vi "RetroParse.vi"(11 "Choose Directory":path) -> ()   [LabVIEW 2022 SP3]
panel:
  out "Raw data":i16[][](graph)
  out "Root Name":string
  out "File num":i32
  in  "Use Selected Files":bool
  in  "Listbox":i32[](listbox)
  in  "file ext":string="000"
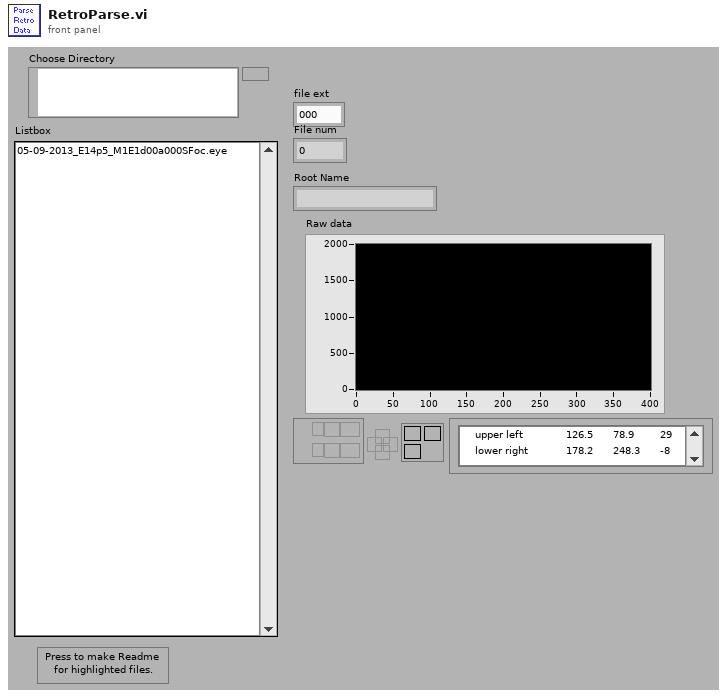
[diagram p1: front panel]
types:
  T1 = enum16{"open", "replace", "create", "open or create", "replace or create", "replace or create with confirmation"}
  T2 = enum16{"big-endian, network order", "native, host order", "little-endian"}
  T3 = typedef "Header.ctl" = cluster{"header info":cluster{"Header":string, "Head length":i16}, "A/D info":cluster{"# rf points per line":u16, "# lines per scan":u16, "sample rate MHz":u16, "# A/D bits":i16, "# bytes per A/D":u16, "TGC Flag":u16, "A/D Type":string}, "Tranducer Info":cluster{"bandwidth":sgl, "center freq":sgl, "start freq":sgl, "ID":i32}, "Scan Info":cluster{"delay":sgl, "pivot distance":sgl, "sector scan angle":sgl, "operator":string, "Scan Mode":string, "location":string}, "Time/Date Info":cluster{"date":string, "time":string}, "RF Info":cluster{"RF file name":string, "RF file att":string, "RF cal file name":string, "RF cal file att":string}, "Patient Info":cluster{"ID":string, "extended ID":string, "age":u16, "sex":string, "previously\nscanned":string, "PSA":sgl, "LOS":u8, "Ethnicty 2":u8, "Race":u8}, "Tissue Type":cluster{"organ":i16, "disease type":i16, "disease location":i16, "IQ_pts":u16, "RcvBuffer":u8, "RcvFrame":u16, "IQBuff":u8, "IQFrame":u16, "IQPage":u8}, "Votage scaling":cluster{"Digitizer (dB)":sgl, "Gain (dB)":sgl, "Atten (dB)":sgl}, "Comment":string, "Misc Info":cluster{"avg num":u16, "c speed":i16, "Div By or SF zones":i16, "XMIT CHS":u8, "RCV CHS":u8, "Xmit angle":sgl}, "Therapy Parameters":cluster{"Theraputic Freq (MHz)":sgl, "Time on (s)":sgl, "Therapy amplitude (mV)":sgl, "Lines Before":u16, "Lines After":u16}, "Scan Settings":cluster{"Energy (uJ or V)":u8, "Damp (Ohm) or Fc":u8, "HP Filt (KHz)":u8, "LP Filt (MHz)":u8, "Gain (db)":u8, "prf (kHz)":sgl, "Distance between\nscan lines (um)":u16, "Distance between\nscan planes (um)":u16, "Scan line gap (um)":sgl, "Scan plane gap (um)":sgl}, "Compression Parameters":cluster{"F1 (MHz)":sgl, "F2 (MHz)":sgl, "% taper":sgl, "duration":sgl}, "Patient Info Xtra":cluster{"First Name":string, "Last Name":string, "Notes":string}, "ROI Box":u16[]}
  T4 = cluster{"Energy (uJ) or V":u8, "Damp (Ohm) or Fc":u8, "HP Filt(KHz) ":u8, "LP Filt (MHz)":u8, "Gain (db)":u8, "prf (kHz)":sgl, "Distance between\nscan lines (mm)":u16, "Distance between\nscan planes (mm)":u16, "Scan line gap (um)":sgl, "Scan plane gap (um)":sgl}
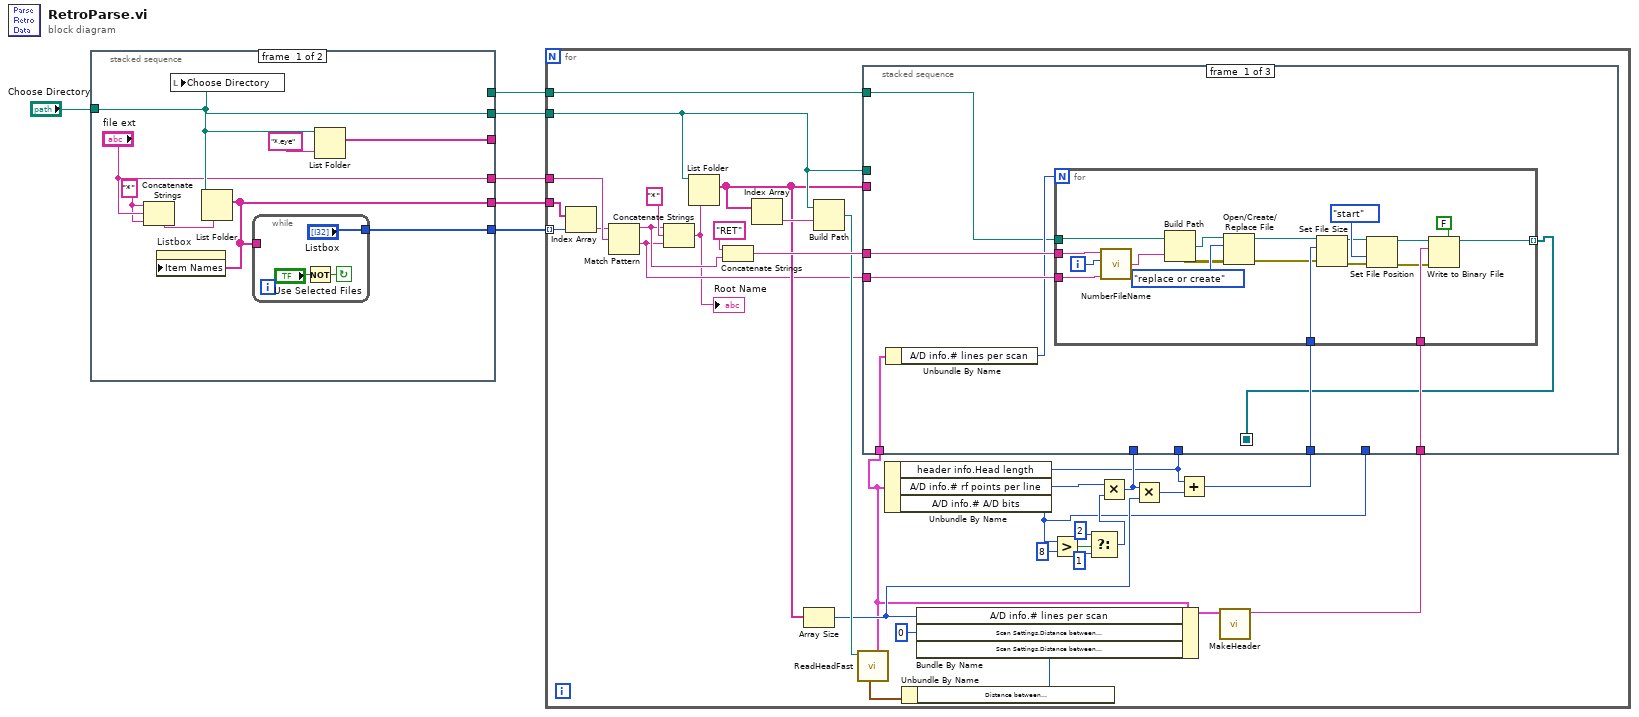
[diagram p0: block diagram]
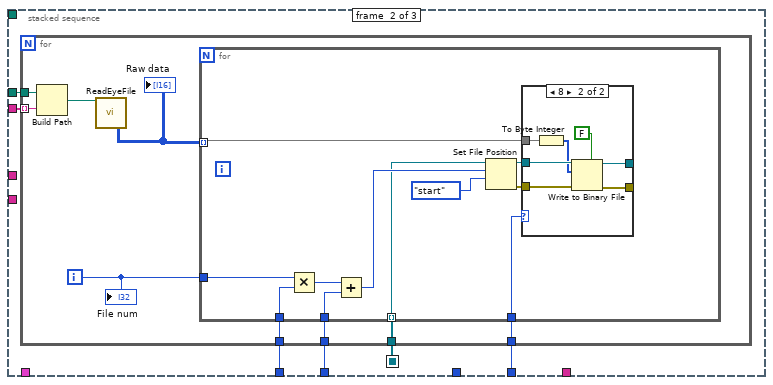
[diagram p2: hidden frame]
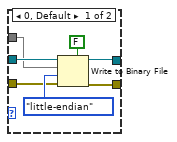
[diagram p3: hidden frame]
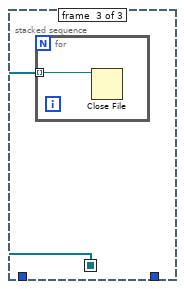
[diagram p4: hidden frame]
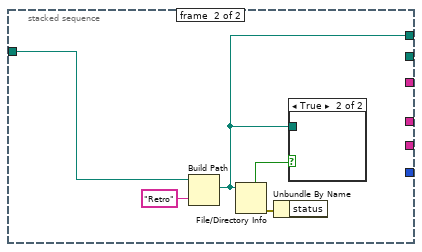
[diagram p5: hidden frame]
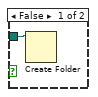
[diagram p6: hidden frame]
diagram:
  n1 = stacked-sequence {
    tunnel: "Choose Directory" -> [w10 w22]
    tunnel: [w13 _] -> _
    tunnel: [w12 _] -> w5
    tunnel: [w11 _] -> w4
    tunnel: ["file ext" _] -> w3
    tunnel: [w10 _] -> w2
    tunnel: [_ w18] -> w1
    frame #0 {
      w7 = "*" ("prompt")
      n2 = Concatenate Strings(w7, "file ext", w7) -> (w8:string)
      n3 = local write "Choose Directory"(w10) -> ()
      n4 = List Folder(path=w10, pattern=w8) -> (filenames=w11:string[])  [unwired: 1 in, 4 out]
      n5 = property on="Listbox" class="LstBox (strict)"("Item Names"=w11) -> ()  [unwired: 2 in, 2 out]
      n6 = while {
        tunnel: ["Listbox"] -> w12
        tunnel: w11 -> [_]
        stop <- w17 continue-if-true
        n7 = Not(x="Use Selected Files") -> (.not. x?=w17:bool)
      }
      n8 = List Folder(path=w10, pattern="*.eye" ("prompt")) -> (filenames=w13:string[])  [unwired: 1 in, 4 out]
    }
    frame #1 {
      n9 = Build Path(base path=w22, name or relative path="Retro") -> (appended path=w18:path)
      n10 = File/Directory Info(path=w18) -> (directory=w20:bool, error out=w19:errorcluster)  [unwired: 1 in, 5 out]
      n11 = Unbundle By Name(w19) -> ()  [unwired: 1 out]
      n12 = case shown="True" w20 {
        tunnel: w18 -> [w23 _]
        frame False {
          n13 = Create Folder(path (use dialog)=w23) -> ()  [unwired: 1 in, 4 out]
        }
        frame True {
        }
      }
    }
  }
  n14 = for {
    tunnel: w5 -> [w55] mode=indexing
    tunnel: w4 -> [w54]
    tunnel: w3 -> [w56]
    tunnel: w2 -> [w47]
    tunnel: w1 -> [w51]
    n15 = Index Array(array=w54, index=w55) -> (element=w53:string)
    n16 = Match Pattern(string=w53, regular expression=w56) -> (before substring=w36:string, after substring=w35:string)  [unwired: 3 out]
    n17 = Concatenate Strings(w36, "*" ("prompt"), w35) -> (w34:string)
    "Root Name" <- w34
    n18 = List Folder(path=w47, pattern=w34) -> (filenames=w45:string[])  [unwired: 1 in, 4 out]
    n19 = Concatenate Strings("RET" ("prompt"), w36) -> (w49:string)
    n20 = Index Array(array=w45) -> (element=w48:string)  [unwired: 1 in]
    n21 = Array Size(array=w45) -> (size(s)=w39:i32)
    n22 = Build Path(base path=w47, name or relative path=w48) -> (appended path=w46:path)
    n23 = call "ReadHeadFast.vi"("new file path"=w46) -> ("Header In"=w33:T3, "Scan Settings (Pulser and Scaping)"=w42:T4)  [unwired: 7 in, 2 out]
    n24 = Unbundle By Name(w33) -> ("header info.Head length"=w26:i16, "A/D info.# rf points per line"=w28:u16, "A/D info.# A/D bits"=w24:i16)
    n25 = Unbundle By Name(w42) -> ("Distance between\nscan planes (mm)"=w41:u16)
    n26 = Bundle By Name(cluster=w33, "A/D info.# lines per scan"=w39, "Scan Settings.Distance between\nscan planes (um)"=u16 0 ("Scan Settings.Distance between\nscan planes (mm)"), "Scan Settings.Distance between\nscan lines (um)"=w41) -> (w44:T3)
    n27 = Greater?(x=w24, y=u16 8) -> (0:w31:bool)
    n28 = Select(t=u16 2 ("y"), s=w31, f=u16 1 ("y")) -> (s? t:f=w29:u16)
    n29 = Multiply(x=w28, y=w29) -> (x*y=w27:u16)
    n30 = Multiply(x=w27, y=w39) -> (x*y=w38:i32)
    n31 = Add(x=w26, y=w38) -> (x+y=w37:i32)
    n32 = call "MakeHeader.vi"("Header In"=w44) -> ("Header String"=w43:string)  [unwired: 6 out]
    n33 = stacked-sequence {
      seq-local: [w60 _ _] -> [_ w83 w123]
      tunnel: w51 -> [w57 _ _]
      tunnel: w49 -> [w61 _ _]
      tunnel: w47 -> [_ w88 _]
      tunnel: w45 -> [_ w87 _]
      tunnel: w43 -> [w64 _ _]
      tunnel: w37 -> [w63 _ _]
      tunnel: w35 -> [w62 _ _]
      tunnel: w33 -> [w59 _ _]
      tunnel: w27 -> [_ w86 _]
      tunnel: w26 -> [_ w85 _]
      tunnel: w24 -> [_ w84 _]
      frame #0 {
        n34 = Unbundle By Name(w59) -> ("A/D info.# lines per scan"=w58:u16)
        n35 = for {
          N: w58 -> [_]
          tunnel: w57 -> [w82]
          tunnel: w61 -> [w78]
          tunnel: w64 -> [w76]
          tunnel: w63 -> [w75]
          tunnel: w62 -> [w74]
          tunnel: [w65] -> w60 mode=indexing
          i -> [w66]
          n36 = call "NumberFileName.vi"("String"=w74, "File number"=w66, "file name"=w78) -> ("Numbered File"=w77:string)  [unwired: 1 in]
          n37 = Build Path(base path=w82, name or relative path=w77) -> (appended path=w81:path)
          n38 = Open/Create/Replace File(file path (use dialog)=w81, operation (0:open)=T1."replace or create") -> (refnum out=w79:refnum<file>, error out=w73:errorcluster)  [unwired: 1 in, 4 out]
          n39 = Set File Size(4:w73, 6:w75, 7:w79) -> (0:w70:errorcluster, 3:w71:refnum<file>)
          n40 = Set File Position(refnum=w71, from (0:start)=enum16{"start", "end", "current"}."start", error in=w70) -> (refnum out=w69:refnum<file>, error out=w68:errorcluster)  [unwired: 1 in]
          n41 = Write to Binary File(file (use dialog)=w69, data=w76, error in=w68, 5:FALSE ("prepend array or string size? (T)")) -> (refnum out=w65:refnum<file>)  [unwired: 4 out]
        }
      }
      frame #1 {
        n42 = for {
          tunnel: w88 -> [w97]
          tunnel: w87 -> [w95] mode=indexing
          tunnel: w86 -> [w92]
          tunnel: w85 -> [w91]
          tunnel: w84 -> [w90]
          tunnel: w83 -> [w89]
          i -> [w94]
          n43 = Build Path(base path=w97, name or relative path=w95) -> (appended path=w96:path)
          n44 = call "ReadEyeFile.vi"("new file path"=w96) -> ("2-D data array"=w93:i16[][])  [unwired: 1 in, 17 out]
          "Raw data" <- w93
          n45 = for {
            tunnel: w93 -> [w108] mode=indexing
            tunnel: w94 -> [w107]
            tunnel: w92 -> [w106]
            tunnel: w91 -> [w104]
            tunnel: w90 -> [w99]
            tunnel: w89 -> [w98] mode=indexing
            n46 = Multiply(x=w107, y=w106) -> (x*y=w105:i32)
            n47 = Add(x=w105, y=w104) -> (x+y=w103:i32)
            n48 = Set File Position(offset (in bytes) (0)=w103, refnum=w98, from (0:start)=enum16{"start", "end", "current"}."start") -> (refnum out=w101:refnum<file>, error out=w100:errorcluster)  [unwired: 1 in]
            n49 = case shown="8" w99 {
              tunnel: w108 -> [w109 w122]
              tunnel: w101 -> [w110 w121]
              tunnel: w100 -> [w111 w120]
              tunnel: [w113 w119] -> _
              tunnel: [w112 w118] -> _
              frame 0, Default {
                n50 = Write to Binary File(file (use dialog)=w110, data=w109, error in=w111, 5:FALSE ("prepend array or string size? (T)"), 9:T2."little-endian" ("byte order (0:big-endian, network order)")) -> (refnum out=w113:refnum<file>, error out=w112:errorcluster)  [unwired: 2 out]
              }
              frame 8 {
                n51 = To Byte Integer(number=w122) -> (8bit integer=w117:i8[])
                n52 = Write to Binary File(file (use dialog)=w121, data=w117, error in=w120, 5:FALSE ("prepend array or string size? (T)")) -> (refnum out=w119:refnum<file>, error out=w118:errorcluster)  [unwired: 1 in, 2 out]
              }
            }
          }
          "File num" <- w94
        }
      }
      frame #2 {
        n53 = for {
          tunnel: w123 -> [w124] mode=indexing
          n54 = Close File(refnum=w124) -> ()  [unwired: 1 in, 2 out]
        }
      }
    }
  }
